vi "viExtractFrame.vi"(0 "input variable":u8[](array[numeric])) -> (1 "FrameSize":u32, 2 "output variable":u8[](array[numeric]))   [LabVIEW 2009]
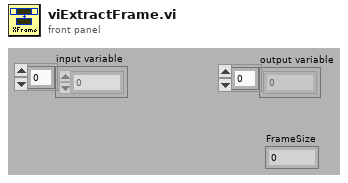
[diagram p1: front panel]
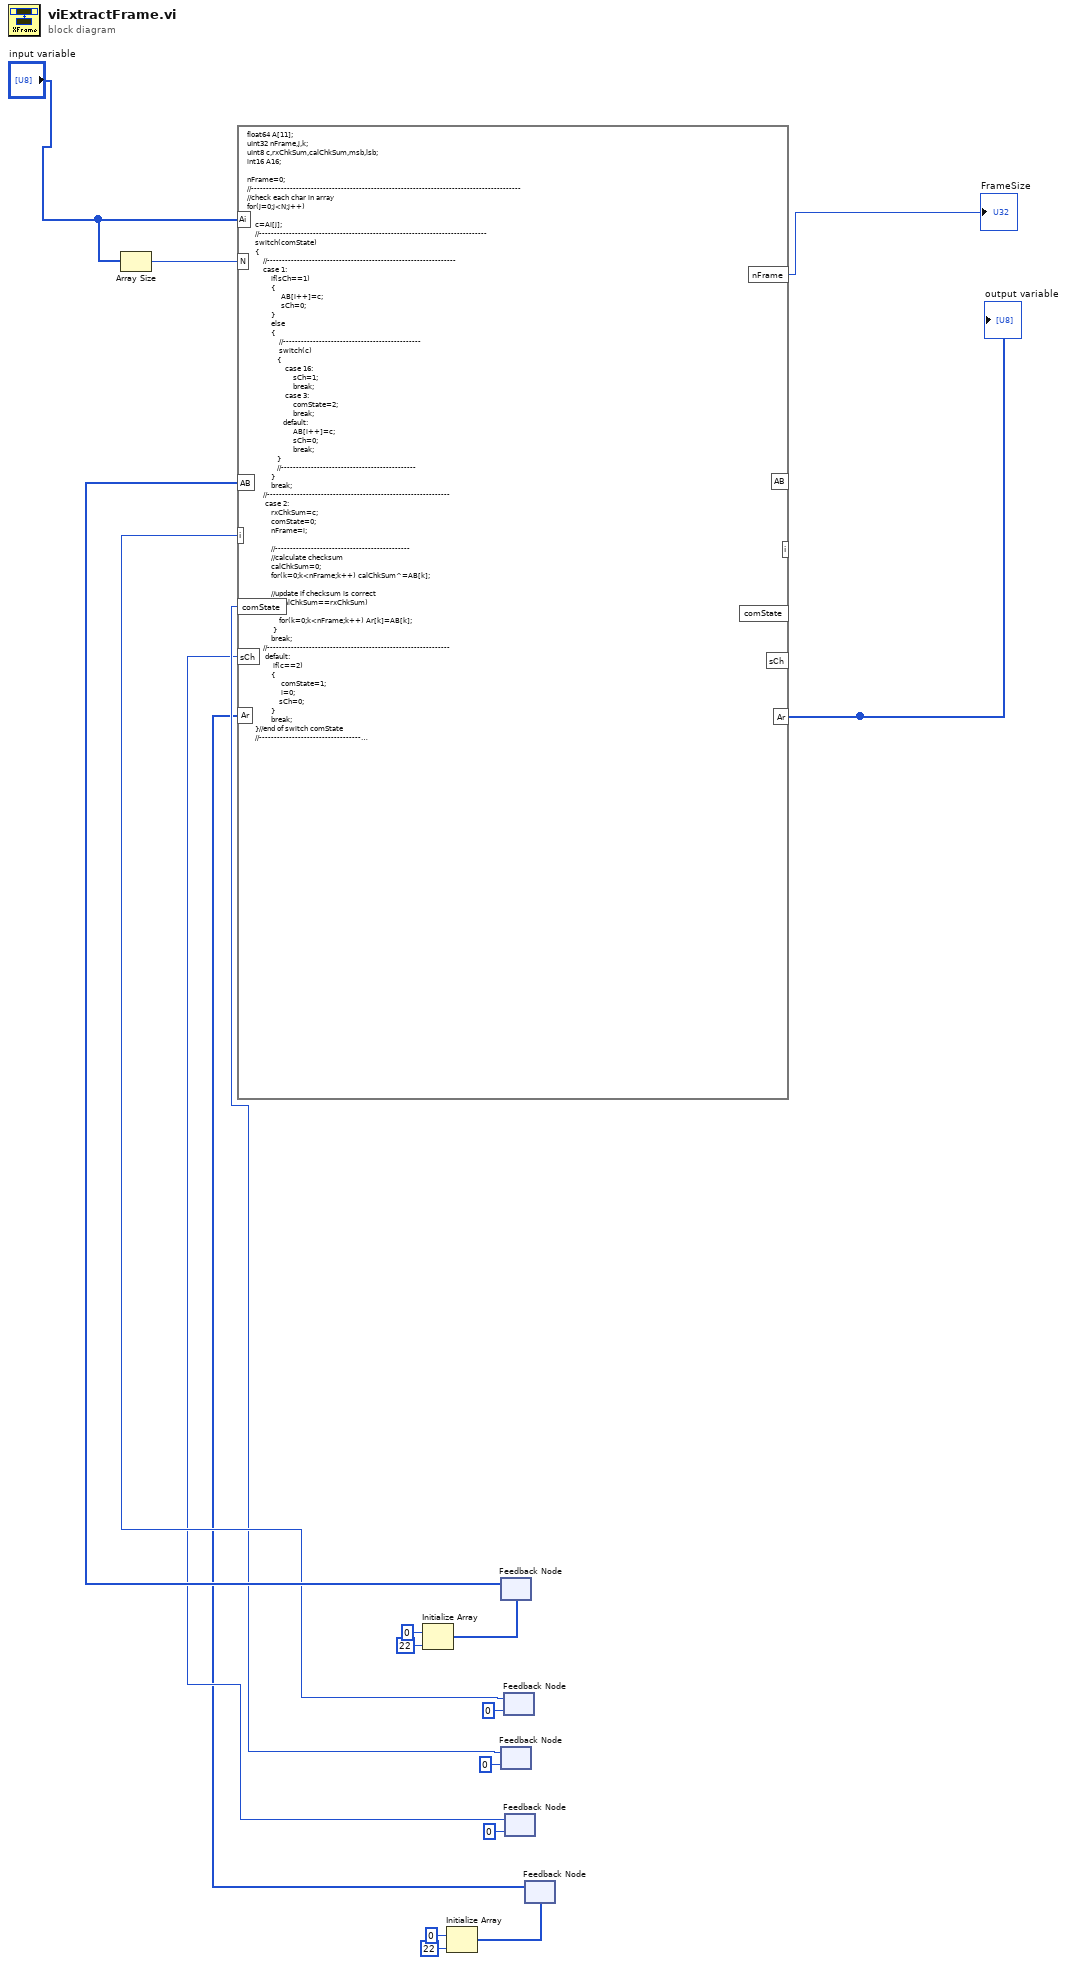
[diagram p0: block diagram]
diagram:
  n1 = Array Size(array="input variable") -> (size(s)=w22:i32)
  n2 = Initialize Array(u8 0 ("element"), 22 ("dimension size")) -> (w17:u8[])
  n3 = Initialize Array(u8 0 ("element"), 22 ("dimension size")) -> (w4:u8[])
  n4 = feedback #1(w17) -> (w21:u8[])
  n5 = feedback #2(u32 0 ("comState")) -> (w8:u32)
  n6 = feedback #3(u32 0 ("i")) -> (w9:u32)
  n7 = feedback #4(u32 0 ("sCh")) -> (w7:u32)
  n8 = feedback #5(w4) -> (w3:u8[])
  n9 = formula code="float64 A[11];\nuInt32 nFrame,j,k;\nuInt8 c,rxChkSum,calChkSum,msb,lsb; \nint16 A16;\n\nnFrame=0;\n//------------------------------------------------------------------------------------------\n//check each char in array\nfor(j=0;j<N;j++)\n{\n    c=Ai[j];\n    //----------------------------------------------------------------------------\n    switch(comState)\n    {\n        //---------------------------------------------------------------\n        case 1:\n            if(sCh==1)\n            {\n                 AB[i++]=c;\n                 sCh=0;\n            }\n            else\n            {\n                //----------------------------------------------\n                switch(c)\n               {\n                   case 16:\n                       sCh=1;\n                       break;\n                   case 3:\n                       comState=2;                      \n                       break;\n                  default:\n                       AB[i++]=c;\n                       sCh=0;\n                       break;\n               }\n               //---------------------------------------------\n            }\n            break;\n        //-------------------------------------------------------------\n         case 2:\n            rxChkSum=c;\n            comState=0;\n            nFrame=i;\n\n            //---------------------------------------------\n            //calculate checksum \n            calChkSum=0;\n            for(k=0;k<nFrame;k++) calChkSum^=AB[k];\n                 \n            //update if checksum is correct\n             if(calChkSum==rxChkSum) \n            {\n                for(k=0;k<nFrame;k++) Ar[k]=AB[k];\n             }           \n            break;\n        //-------------------------------------------------------------\n         default:\n             if(c==2)\n            {\n                 comState=1;               \n                 i=0;\n                sCh=0;                \n            }\n            break;\n    }//end of switch comState  \n    //--------------------------------------------------------------------------\n}//end of for j\n//------------------------------------------------------------------------------------------"("Ai"="input variable", "N"=w22, "AB"=w21, "comState"=w8, "sCh"=w7, "i"=w9, "Ar"=w3) -> ("AB"=w20:u8[], "nFrame"=→"FrameSize":u32, "i"=w15:u32, "comState"=w13:u32, "sCh"=w11:u32, "Ar"=w2:u8[])
  "output variable" <- w2
